vi "StdRowHeightGlobal.vi"() -> ()   [LabVIEW 2013]
panel:
  in  "StdRowHeight":u32=15
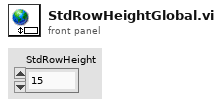
[diagram p1: front panel]
diagram:
